vi "LNLS Control Receive Command Header.vi"(8 "error in (no error)":errorcluster, 10 "timeout ms (10000)":i32=10000, 11 "connection ID":refnum<k5>) -> (0 "error out":errorcluster, 2 "command ID":u8, 3 "connection ID out":refnum<k5>)   [LabVIEW 2011, in "LNLS Control VIs.lvlib"]
uses:
  LNLS Control VIs.lvlib
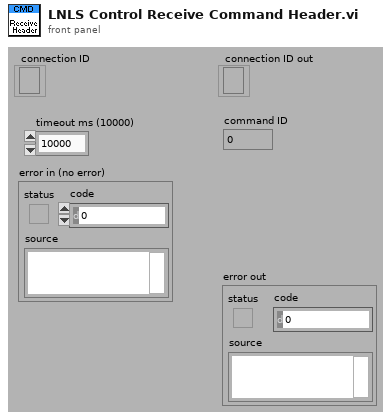
[diagram p1: front panel]
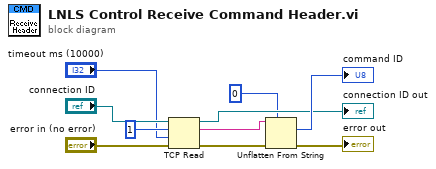
[diagram p0: block diagram]
diagram:
  n1 = TCP Read(connection ID="connection ID", bytes to read=1, error in (no error)="error in (no error)", 9:"timeout ms (10000)") -> (connection ID out=→"connection ID out":refnum<k5>, data out=w1:string, error out=w7:errorcluster)  [unwired: 1 in]
  n2 = Unflatten From String(type=u8 0 ("length"), binary string=w1, error in (no error)=w7) -> (value=→"command ID":u8, error out=→"error out":errorcluster)  [unwired: 2 in, 1 out]
